vi "read_access_codes_from_file.vi"(8 "error in (no error)":errorcluster, 11 "Path":path) -> (0 "error out":errorcluster, 3 "Codes":T1)   [LabVIEW 2016]
uses:
  <vilib>/Utility/config.llb/Read Key (String).vi
  <vilib>/Utility/config.llb/NI_LVConfig.lvlib
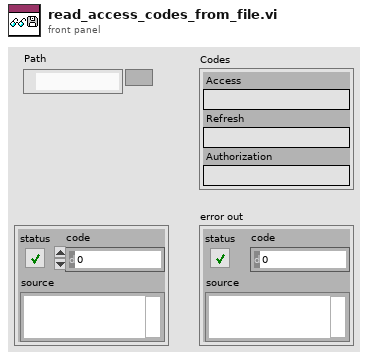
[diagram p1: front panel]
types:
  T1 = cluster{"Access":string, "Refresh":string, "Authorization":string}
  T2 = typedef "NI_LVConfig.lvlib/Config Data RefNum.ctl" = refnum<k1>
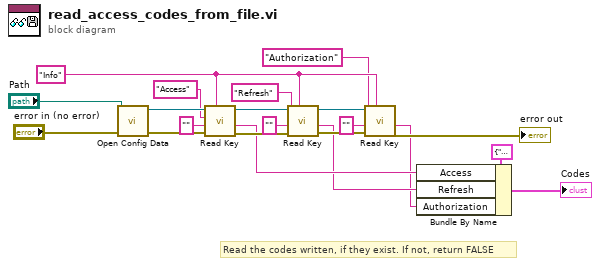
[diagram p0: block diagram]
diagram:
  w7 = "Info"
  # "Read the codes written, if they exist. If not, return FALSE"
  n1 = call <vilib>:"Open Config Data.vi"("error in (no error)"="error in (no error)", "configuration file path"="Path") -> ("error out"=w16:errorcluster, "refnum"=w20:T2)  [unwired: 7 in, 1 out]
  n2 = call-poly <vilib>:"Read Key.vi"("section"=w7, "error in (no error)"=w16, "default value"="", "key"="Access", "refnum"=w20) -> ("error out"=w15:errorcluster, "value"=w10:string, "refnum out"=w19:T2)  [unwired: 3 in, 1 out]
  n3 = call-poly <vilib>:"Read Key.vi"("section"=w7, "error in (no error)"=w15, "default value"="", "key"="Refresh", "refnum"=w19) -> ("error out"=w14:errorcluster, "value"=w9:string, "refnum out"=w18:T2)  [unwired: 3 in, 1 out]
  n4 = call-poly <vilib>:"Read Key.vi"("section"=w7, "error in (no error)"=w14, "default value"="", "key"="Authorization", "refnum"=w18) -> ("error out"=→"error out":errorcluster, "value"=w8:string)  [unwired: 3 in, 2 out]
  n5 = Bundle By Name(cluster=T1 {"Access"="", "Refresh"="", "Authorization"=""}, "Access"=w10, "Refresh"=w9, "Authorization"=w8) -> (→"Codes":T1)
